vi "sub_4610_main.vi"(8 "error in":errorcluster) -> (0 "error out":errorcluster)   [LabVIEW 2019]
uses:
  _ctrl/create-rw-close.ctl
  _ctrl/BP4610_cmd.ctl
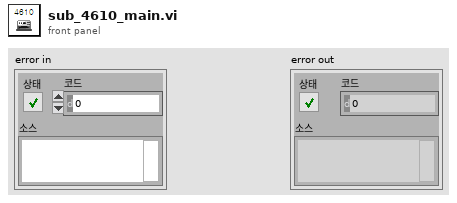
[diagram p1: front panel]
types:
  T1 = typedef "create-rw-close.ctl" = enum16{"create", "write", "read", "delete", "close"}
  T2 = typedef "BP4610_cmd.ctl" = enum16{"open", "read", "set", "set_seq", "limit", "limit_seq", "output on", "output off", "close"}
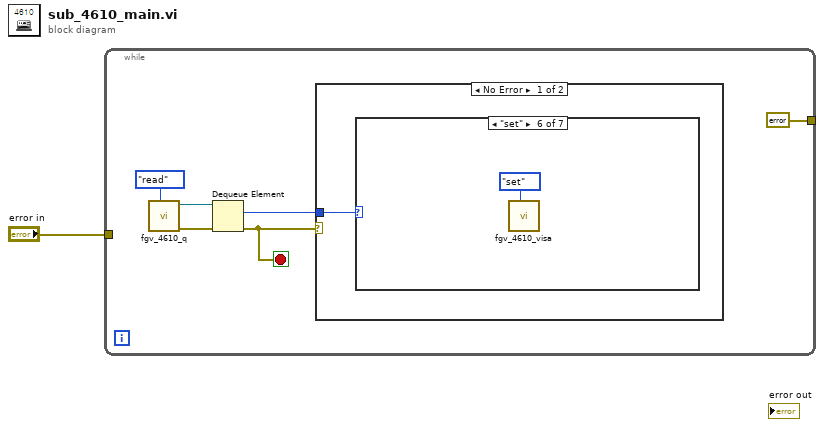
[diagram p0: block diagram]
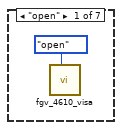
[diagram p2: hidden frame]
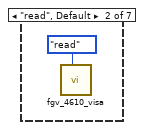
[diagram p3: hidden frame]
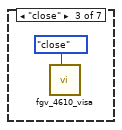
[diagram p4: hidden frame]
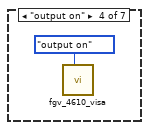
[diagram p5: hidden frame]
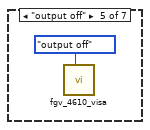
[diagram p6: hidden frame]
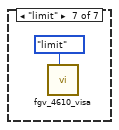
[diagram p7: hidden frame]
diagram:
  n1 = while {
    tunnel: [errorcluster {"status"=FALSE, "code"=0, "source"=""} ("error out")] -> _
    tunnel: "error in" -> [_]
    stop <- w3 stop-if-true
    n2 = call "fgv_4610_q.vi"("cmd"=create-rw-close."read") -> ("error out"=w6:errorcluster, "queue out"=w5:refnum<queue>)  [unwired: 9 in]
    n3 = Dequeue Element(queue=w5, error in (no error)=w6) -> (element=w4:T2, error out=w3:errorcluster)  [unwired: 1 in, 2 out]
    n4 = case shown="No Error" w3 {
      tunnel: w4 -> [w8 _]
      frame No Error {
        n5 = case shown="\"set\"" w8 {
          frame "open" {
            n6 = call "fgv_4610_visa.vi"("cmd"=BP4610_cmd."open") -> ()  [unwired: 10 in, 1 out]
          }
          frame "read", Default {
            n7 = call "fgv_4610_visa.vi"("cmd"=BP4610_cmd."read") -> ()  [unwired: 10 in, 1 out]
          }
          frame "close" {
            n8 = call "fgv_4610_visa.vi"("cmd"=BP4610_cmd."close") -> ()  [unwired: 10 in, 1 out]
          }
          frame "output on" {
            n9 = call "fgv_4610_visa.vi"("cmd"=BP4610_cmd."output on") -> ()  [unwired: 10 in, 1 out]
          }
          frame "output off" {
            n10 = call "fgv_4610_visa.vi"("cmd"=BP4610_cmd."output off") -> ()  [unwired: 10 in, 1 out]
          }
          frame "set" {
            n11 = call "fgv_4610_visa.vi"("cmd"=BP4610_cmd."set") -> ()  [unwired: 10 in, 1 out]
          }
          frame "limit" {
            n12 = call "fgv_4610_visa.vi"("cmd"=BP4610_cmd."limit") -> ()  [unwired: 10 in, 1 out]
          }
        }
      }
      frame Error {
      }
    }
  }
